vi "New - Update Poly Set Map.vi"(6 "Instance Info":T1={"VIPath"=path "C:/Projects/GitHub/data-record-ad-internal/Data Types/ADAS Generic/Read.vi", "Menu Name"="Generic", "Selector Name"="Generic"}, 10 "Poly VI Name in":string, 11 "Poly Map Set in":T2) -> (2 "Poly VI Name out":string, 3 "Poly Map Set out":T2)   [LabVIEW 2020]
uses:
  _td_cluster_InstanceInfo.ctl
  _td_map_PolyInstanceInfo.ctl
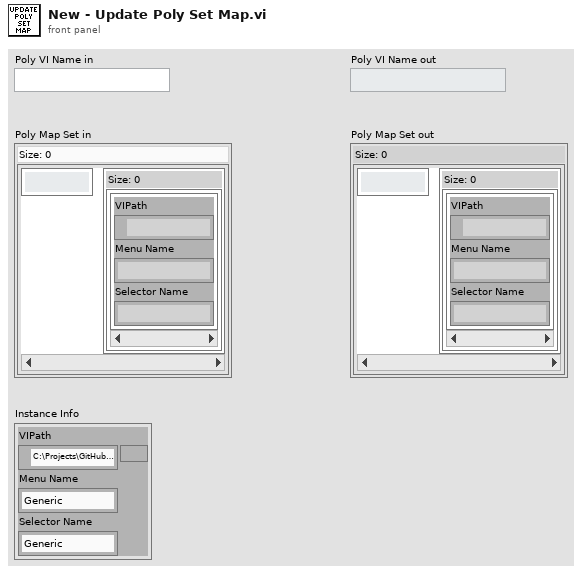
[diagram p1: front panel]
types:
  T1 = typedef "_td_cluster_InstanceInfo.ctl" = cluster{"VIPath":path, "Menu Name":string, "Selector Name":string}
  T2 = typedef "_td_map_PolyInstanceInfo.ctl" = map{string, set{T1}}
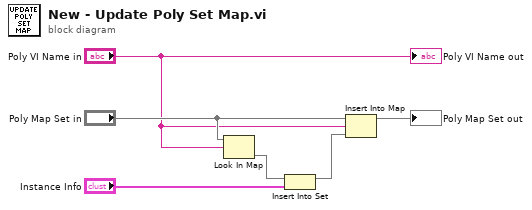
[diagram p0: block diagram]
diagram:
  n1 = Look In Map(map="Poly Map Set in", key="Poly VI Name in") -> (value=w6:set{T1})  [unwired: 1 in, 1 out]
  n2 = Insert Into Set(10:"Instance Info", 11:w6) -> (3:w5:set{T1})  [unwired: 1 out]
  n3 = Insert Into Map(map in="Poly Map Set in", key="Poly VI Name in", value=w5) -> (map out=→"Poly Map Set out":T2)  [unwired: 2 out]
  "Poly VI Name out" <- "Poly VI Name in"
